vi "Get Content Bounds.vi"(0 "Array":bool[][](array[boolean])) -> (1 "Start (Inclusive)":i32[](array[numeric]), 2 "End  (Inclusive)":i32[](array[numeric]), 3 "Size":i32[](array[numeric]))   [LabVIEW 2020, in "VIM Tools.lvlib"]
uses:
  VIM Tools.lvlib
  6e0c4393-7d25-453f-9138-b502b35675a0.vi
  5a7323a8-862b-4b00-8fbf-75c78e518ac2.vi
  3c6a847f-080a-415b-8244-8488da89b8b9.vi
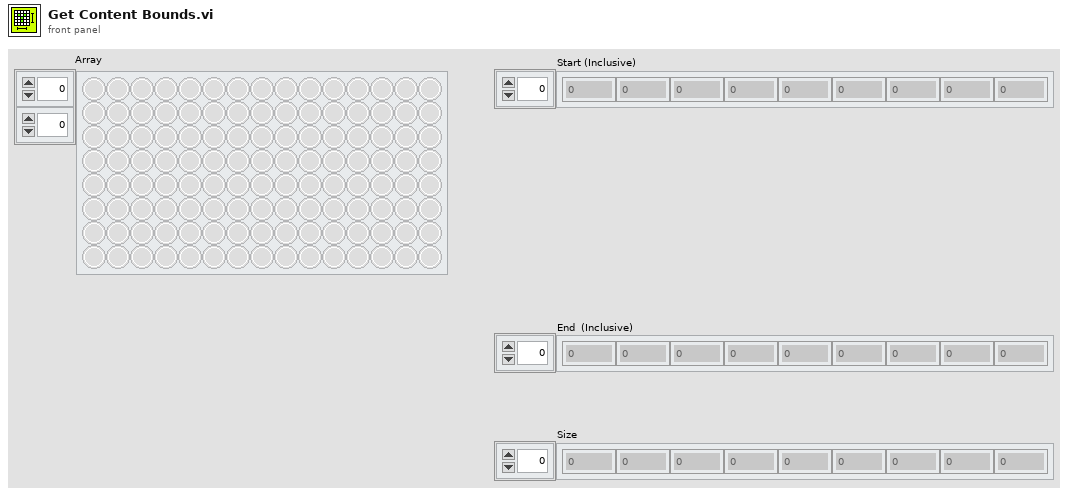
[diagram p1: front panel]
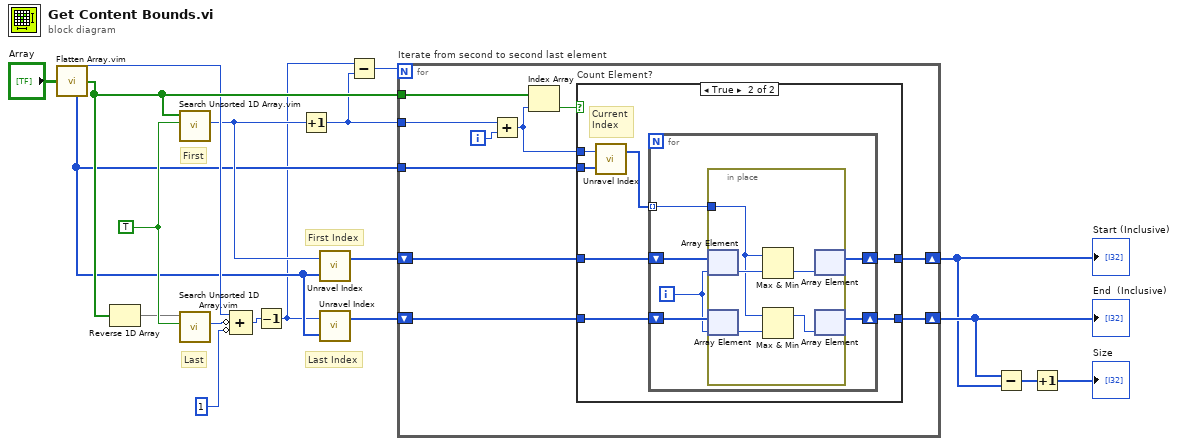
[diagram p0: block diagram]
diagram:
  w17 = TRUE
  # "Last Index"
  # "First Index"
  # "First"
  # "Last"
  n1 = call "Flatten Array.vim"("ND Array In"="Array") -> ("New Size"=w15:i32, "1D Array out"=w18:bool[], "Old Size"=w11:i32[])  [unwired: 6 in]
  n2 = Reverse 1D Array(array=w18) -> (reversed array=w16:bool[])
  n3 = call "Search Unsorted 1D Array.vim"("element"=w17, "unsorted 1D array"=w18) -> ("index of element"=w13:i32)  [unwired: 9 in]
  n4 = call "Search Unsorted 1D Array.vim"("element"=w17, "unsorted 1D array"=w16) -> ("index of element"=w14:i32)  [unwired: 9 in]
  n5 = Compound Arithmetic op=ADD(w15, invert w14, invert 1 ("value")) -> (w4:i32)
  n6 = Decrement(x=w4) -> (x-1=w3:i32)
  n7 = Increment(x=w13) -> (x+1=w2:i32)
  n8 = call "Unravel Index.vi"("shape"=w11, "Flat Index"=w13) -> ("ND Index"=w12:i32[])  [unwired: 1 out]
  n9 = call "Unravel Index.vi"("shape"=w11, "Flat Index"=w3) -> ("ND Index"=w10:i32[])  [unwired: 1 out]
  n10 = Subtract(x=w3, y=w2) -> (x-y=w9:i32)
  n11 = for "Iterate from second to second last element" {
    N: w9 -> [_]
    tunnel: w18 -> [w25]
    tunnel: w11 -> [w28]
    tunnel: w2 -> [w27]
    shift-right: [w26] -> w7
    shift-left: w12 -> [w23]
    shift-right: [w21] -> w8
    shift-left: w10 -> [w22]
    i -> [w29]
    n12 = Add(x=w27, y=w29) -> (x+y=w24:i32)
    n13 = Index Array(array=w25, index=w24) -> (element=w20:bool)
    n14 = case "Count Element?" shown="True" w20 {
      tunnel: w28 -> [_ w38]
      tunnel: w24 -> [_ w37]
      tunnel: [w30 w34] -> w26
      tunnel: w23 -> [w30 w36]
      tunnel: w22 -> [w31 w35]
      tunnel: [w31 w33] -> w21
      frame False {
      }
      frame True {
        # "Current\nIndex"
        n15 = call "Unravel Index.vi"("shape"=w38, "Flat Index"=w37) -> ("ND Index"=w32:i32[])  [unwired: 1 out]
        n16 = for {
          tunnel: w32 -> [w40] mode=indexing
          shift-right: [w43] -> w34
          shift-left: w36 -> [w44]
          shift-right: [w39] -> w33
          shift-left: w35 -> [w42]
          i -> [w41]
          n17 = in-place {
            in-place-border: w40 -> [w47]
            n18 = in-place-array #1(w44, w41) -> (w49:i32)
            n19 = in-place-array #2(w42, w41) -> (w46:i32)
            n20 = Max & Min(x=w47, y=w49) -> (min(x,y)=w48:i32)  [unwired: 1 out]
            n21 = Max & Min(x=w47, y=w46) -> (max(x,y)=w45:i32)  [unwired: 1 out]
            n22 = in-place-array #1(w48) -> (w43:i32[])  [unwired: 1 out]
            n23 = in-place-array #2(w45) -> (w39:i32[])  [unwired: 1 out]
          }
        }
      }
    }
  }
  "Start (Inclusive)" <- w7
  "End  (Inclusive)" <- w8
  n24 = Subtract(x=w8, y=w7) -> (x-y=w6:i32[])
  n25 = Increment(x=w6) -> (x+1=→"Size":i32[])
